vi "Parse.vi"(8 "error in (no error)":errorcluster, 11 "TransformTokenizer in":refnum<class "TransformTokenizer.lvclass">) -> (0 "error out":errorcluster, 3 "TransformTokenizer out":refnum<class "TransformTokenizer.lvclass">)   [LabVIEW 2019, in "TransformTokenizer.lvclass"]
uses:
  TransformTokenizer.lvclass
  TransformTokenizer.lvclass/TransformTokenizer.ctl
  States.ctl
panel:
  out "Array":string[](array[string])
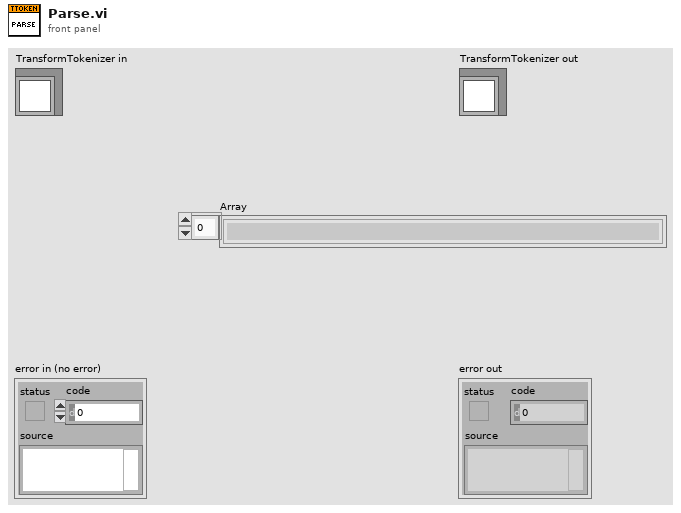
[diagram p1: front panel]
types:
  T1 = typedef "TransformTokenizer.lvclass/States.ctl" = enum16{"Is End", "Exit", "Get Transform", "Get Type", "Get Coords"}
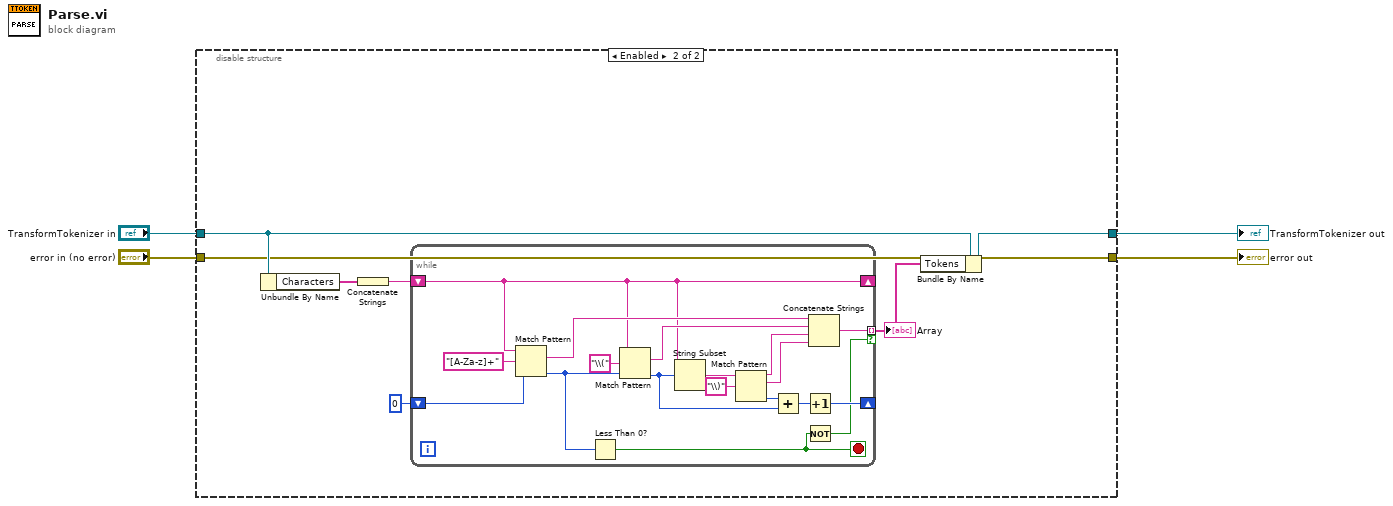
[diagram p0: block diagram]
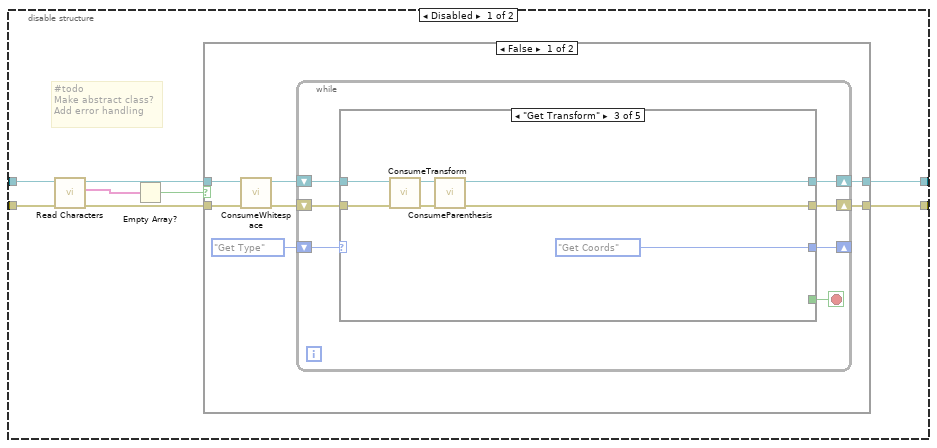
[diagram p2: hidden frame]
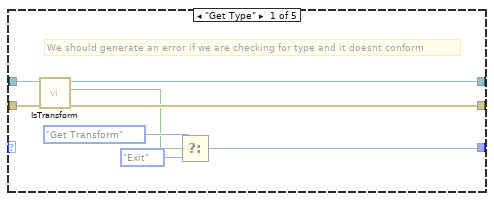
[diagram p3: hidden frame]
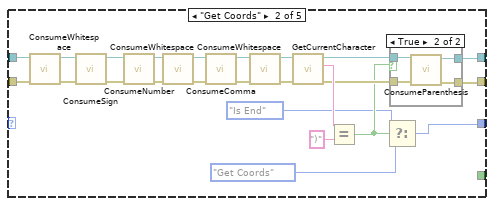
[diagram p4: hidden frame]
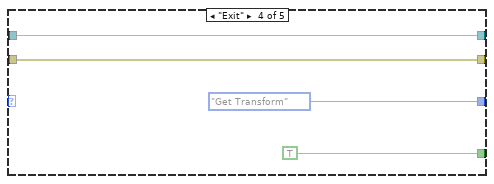
[diagram p6: hidden frame]
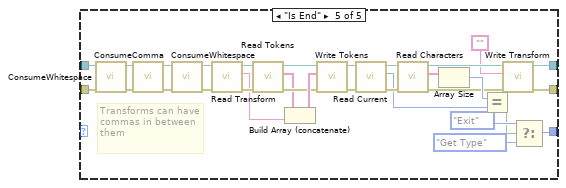
[diagram p7: hidden frame]
diagram:
  n1 = disable-structure shown="Enabled" {
    disable-tunnel: [w12 w109] -> w4
    disable-tunnel: [w11 w110] -> w3
    disable-tunnel: "error in (no error)" -> [w10 w109]
    disable-tunnel: "TransformTokenizer in" -> [w8 w112]
    frame Disabled {
      # "#todo\nMake abstract class?\nAdd error handling"
      n2 = call "Read Characters.vi"("error in (no error)"=w10, "TransformTokenizer in"=w8) -> ("error out"=w9:errorcluster, "Characters"=w5:string[], "TransformTokenizer out"=w7:refnum<class "TransformTokenizer.lvclass">)  [unwired: 7 in]
      n3 = Empty Array?(array=w5) -> (empty?=w6:bool)
      n4 = case shown="False" w6 {
        tunnel: [w17 w107] -> w12
        tunnel: [w15 w108] -> w11
        tunnel: w9 -> [w14 w107]
        tunnel: w7 -> [w13 w108]
        frame False {
          n5 = call "ConsumeWhitespace.vi"("error in (no error)"=w14, "TransformTokenizer in"=w13) -> ("error out"=w18:errorcluster, "TransformTokenizer out"=w19:refnum<class "TransformTokenizer.lvclass">)  [unwired: 8 in]
          n6 = while {
            shift-right: [w23] -> w15
            shift-left: w19 -> [w26]
            shift-right: [w24] -> w17
            shift-left: w18 -> [w25]
            shift-right: [w21] -> _
            shift-left: States."Get Type" -> [w22]
            stop <- w20 stop-if-true
            n7 = case shown="\"Get Transform\"" w22 {
              tunnel: w26 -> [w33 w56 w70 w74 w106]
              tunnel: w25 -> [w32 w58 w69 w75 w105]
              tunnel: [w31 w37 w67 w75 w85] -> w24
              tunnel: [w34 w39 w68 w74 w84] -> w23
              tunnel: [w30 w41 States."Get Coords" States."Get Transform" w100] -> w21
              tunnel: [_ _ _ TRUE _] -> w20
              frame "Get Type" {
                # "We should generate an error if we are checking for type and it doesnt conform"
                n8 = call "IsTransform.vi"("error in (no error)"=w32, "TransformTokenizer in"=w33) -> ("error out"=w31:errorcluster, "Transform?"=w27:bool, "TransformTokenizer out"=w34:refnum<class "TransformTokenizer.lvclass">)  [unwired: 7 in]
                n9 = Select(t=States."Get Transform", s=w27, f=States."Exit") -> (s? t:f=w30:T1)
              }
              frame "Get Coords" {
                n10 = call "ConsumeWhitespace.vi"("error in (no error)"=w58, "TransformTokenizer in"=w56) -> ("error out"=w55:errorcluster, "TransformTokenizer out"=w57:refnum<class "TransformTokenizer.lvclass">)  [unwired: 8 in]
                n11 = call "ConsumeSign.vi"("error in (no error)"=w55, "TransformTokenizer in"=w57) -> ("error out"=w53:errorcluster, "TransformTokenizer out"=w54:refnum<class "TransformTokenizer.lvclass">)  [unwired: 8 in]
                n12 = call "ConsumeNumber.vi"("error in (no error)"=w53, "TransformTokenizer in"=w54) -> ("error out"=w51:errorcluster, "TransformTokenizer out"=w52:refnum<class "TransformTokenizer.lvclass">)  [unwired: 8 in]
                n13 = call "ConsumeWhitespace.vi"("error in (no error)"=w51, "TransformTokenizer in"=w52) -> ("error out"=w49:errorcluster, "TransformTokenizer out"=w50:refnum<class "TransformTokenizer.lvclass">)  [unwired: 8 in]
                n14 = call "ConsumeComma.vi"("error in (no error)"=w49, "TransformTokenizer in"=w50) -> ("error out"=w47:errorcluster, "TransformTokenizer out"=w48:refnum<class "TransformTokenizer.lvclass">)  [unwired: 8 in]
                n15 = call "ConsumeWhitespace.vi"("error in (no error)"=w47, "TransformTokenizer in"=w48) -> ("error out"=w45:errorcluster, "TransformTokenizer out"=w46:refnum<class "TransformTokenizer.lvclass">)  [unwired: 8 in]
                n16 = call "GetCurrentCharacter.vi"("error in (no error)"=w45, "TransformTokenizer in"=w46) -> ("error out"=w38:errorcluster, "Character"=w44:string, "TransformTokenizer out"=w40:refnum<class "TransformTokenizer.lvclass">)  [unwired: 7 in]
                n17 = Equal?(x=w44, y=")") -> (x = y?=w36:bool)
                n18 = Select(t=States."Is End", s=w36, f=States."Get Coords") -> (s? t:f=w41:T1)
                n19 = case shown="True" w36 {
                  tunnel: w40 -> [w59 w64]
                  tunnel: [w59 w63] -> w39
                  tunnel: w38 -> [w60 w62]
                  tunnel: [w60 w61] -> w37
                  frame False {
                  }
                  frame True {
                    n20 = call "ConsumeParenthesis.vi"("error in (no error)"=w62, "TransformTokenizer in"=w64) -> ("error out"=w61:errorcluster, "TransformTokenizer out"=w63:refnum<class "TransformTokenizer.lvclass">)  [unwired: 8 in]
                  }
                }
              }
              frame "Get Transform" {
                n21 = call "ConsumeTransform.vi"("error in (no error)"=w69, "TransformTokenizer in"=w70) -> ("error out"=w65:errorcluster, "TransformTokenizer out"=w66:refnum<class "TransformTokenizer.lvclass">)  [unwired: 8 in]
                n22 = call "ConsumeParenthesis.vi"("error in (no error)"=w65, "TransformTokenizer in"=w66) -> ("error out"=w67:errorcluster, "TransformTokenizer out"=w68:refnum<class "TransformTokenizer.lvclass">)  [unwired: 8 in]
              }
              frame "Exit" {
              }
              frame "Is End" {
                # "Transforms can have commas in between them"
                n23 = call "ConsumeWhitespace.vi"("error in (no error)"=w105, "TransformTokenizer in"=w106) -> ("error out"=w80:errorcluster, "TransformTokenizer out"=w81:refnum<class "TransformTokenizer.lvclass">)  [unwired: 8 in]
                n24 = call "ConsumeComma.vi"("error in (no error)"=w80, "TransformTokenizer in"=w81) -> ("error out"=w77:errorcluster, "TransformTokenizer out"=w79:refnum<class "TransformTokenizer.lvclass">)  [unwired: 8 in]
                n25 = call "ConsumeWhitespace.vi"("error in (no error)"=w77, "TransformTokenizer in"=w79) -> ("error out"=w76:errorcluster, "TransformTokenizer out"=w78:refnum<class "TransformTokenizer.lvclass">)  [unwired: 8 in]
                n26 = call "Read Transform.vi"("error in (no error)"=w76, "TransformTokenizer in"=w78) -> ("error out"=w88:errorcluster, "Transform"=w87:string, "TransformTokenizer out"=w89:refnum<class "TransformTokenizer.lvclass">)  [unwired: 7 in]
                n27 = call "Read Tokens.vi"("error in (no error)"=w88, "TransformTokenizer in"=w89) -> ("error out"=w91:errorcluster, "Transforms"=w90:string[], "TransformTokenizer out"=w92:refnum<class "TransformTokenizer.lvclass">)  [unwired: 7 in]
                n28 = Build Array (concatenate)(w90, w87) -> (w93:string[])
                n29 = call "Write Tokens.vi"("error in (no error)"=w91, "Transforms"=w93, "TransformTokenizer in"=w92) -> ("error out"=w94:errorcluster, "TransformTokenizer out"=w95:refnum<class "TransformTokenizer.lvclass">)  [unwired: 7 in]
                n30 = call "Read Current.vi"("error in (no error)"=w94, "TransformTokenizer in"=w95) -> ("error out"=w103:errorcluster, "Current"=w101:i32, "TransformTokenizer out"=w104:refnum<class "TransformTokenizer.lvclass">)  [unwired: 7 in]
                n31 = call "Read Characters.vi"("error in (no error)"=w103, "TransformTokenizer in"=w104) -> ("error out"=w86:errorcluster, "Characters"=w102:string[], "TransformTokenizer out"=w83:refnum<class "TransformTokenizer.lvclass">)  [unwired: 7 in]
                n32 = Array Size(array=w102) -> (size(s)=w96:i32)
                n33 = Equal?(x=w96, y=w101) -> (x = y?=w98:bool)
                n34 = call "Write Transform.vi"("error in (no error)"=w86, "Transform"="", "TransformTokenizer in"=w83) -> ("error out"=w85:errorcluster, "TransformTokenizer out"=w84:refnum<class "TransformTokenizer.lvclass">)  [unwired: 7 in]
                n35 = Select(t=States."Exit", s=w98, f=States."Get Type") -> (s? t:f=w100:T1)
              }
            }
          }
        }
        frame True {
        }
      }
    }
    frame Enabled {
      n36 = Unbundle By Name(w112) -> ("Characters"=w115:string[])
      n37 = Concatenate Strings(w115) -> (w114:string)
      n38 = while {
        shift-right: [w119] -> _
        shift-left: w114 -> [w119]
        shift-right: [w122] -> _
        shift-left: 0 -> [w121]
        tunnel: [w117] -> w111 mode=indexing if=w116
        stop <- w118 stop-if-true
        n39 = Match Pattern(string=w119, regular expression="[A-Za-z]+", offset (0)=w121) -> (match substring=w130:string, offset past match=w120:i32)  [unwired: 2 out]
        n40 = Less Than 0?(x=w120) -> (x < 0?=w118:bool)
        n41 = Match Pattern(string=w119, regular expression="\\(", offset (0)=w120) -> (match substring=w128:string, offset past match=w124:i32)  [unwired: 2 out]
        n42 = String Subset(string=w119, offset (0)=w124) -> (substring=w127:string)  [unwired: 1 in]
        n43 = Match Pattern(string=w127, regular expression="\\)") -> (before substring=w126:string, match substring=w129:string, offset past match=w125:i32)  [unwired: 1 in, 1 out]
        n44 = Add(x=w125, y=w124) -> (x+y=w123:i32)
        n45 = Increment(x=w123) -> (x+1=w122:i32)
        n46 = Not(x=w118) -> (.not. x?=w116:bool)
        n47 = Concatenate Strings(w130, w128, w126, w129) -> (w117:string)
      }
      "Array" <- w111
      n48 = Bundle By Name(cluster=w112, "Tokens"=w111) -> (w110:refnum<class "TransformTokenizer.lvclass">)
    }
  }
  "error out" <- w4
  "TransformTokenizer out" <- w3
